vi "Pulse Measurement.vi"(0 "session":T3={"3620 session"=refnum, "tx baseband session"={"3610 session"={"VISA resource name"="", "Address Space"=1, "window_offset"=0, "register_addresses"={"MM based Registers"={"Revision"=0, "OldestCompatRev"=0, "signature"=0, "scratch"=0, "LedControl"=0, "BoardHwRev"=0, "BoardControl"=0, "ThermalStatus"=0, "BasebandStatus"=0, "BasebandControl"=0, "BasebandAuxSetup"=0, "BasebandAuxStatus"=0, "LmkSyncOutSetup"=0, " AdcSyncOutSetup"=0, " InjSyncOutSetup"=0, " PxiTrig0OutSetup"=0, " PxiTrig1OutSetup"=0, " PxiTrig2OutSetup"=0, " PxiTrig3OutSetup"=0, " PxiTrig4OutSetup"=0, " PxiTrig5OutSetup"=0, " PxiTrig6OutSetup"=0, " PxiTrig7OutSetup"=0}, "CPLD based Registers"={"SlaveSignature"=0, "SlaveRevision"=0, "SlaveOldestCompatRev"=0, "SlaveScratch"=0, "SlaveSetup"=0, "SlaveStatus"=0, "IDacReg_offset"=0, "LMKRegGrp0_offset"=0, "QDacReg_offset"=0, "BrdTempSensorVal"=0, "TempSensorPowerDown"=0, "GPIOReg_offset"=0, "IAdcReg_offset"=0, "QAdcReg_offset"=0, "LMKRegGrp1_offset"=0, "QadcTempSensorVal"=0, "IadcTempSensorVal"=0, "RevisionReg"=0, "VcxoReg"=0, "CpldStatusReg"=0, "PowerReg"=0, "VBiasEnReg"=0, "ExtRefOeReg"=0, "QdacCtrlReg"=0, "QdacStatusReg"=0, "IdacCtrlReg"=0, "IdacStatusReg"=0, "QdacJtagIn"=0, "QdacJtagOut"=0, "IdacJtagIn"=0, "IdacJtagOut"=0, "IqDcSetupReg"=0, "QadcStatusReg"=0, "IadcStatusReg"=0, "BrdSetupReg"=0, "IqDcRevisionReg"=0, "PllStatusReg"=0, "EndpointScratchReg"=0, "AdcSyncCfgReg"=0, "IqCardOpampReg"=0}, "CPLD Register Offset"=0, "MM  Register Offset"=0, " PxiTrig0OutSetup"=0}, "required_MM_fpga_version"={"signature"=0, "hardware"=0, "current revision"=0, "oldest revision"=0}, "CPLD Oldest Compat Version "={"hardware"=0, "CPLD firmware"=0}, "MM_FPGA_image_location"="", "is_init"=FALSE, "card_type"=enum."ADC", "DacLmkConfigFileName"="", "AdcLmkConfigFileName"="", "AdcConfigFileName"="", "DacConfigFileName_RevA"="", "DacConfigFileName_RevB"="", "Mulde hardware revision"=0, "bypass DAC PLL\n"=FALSE, "IQ Card Revision"=enum."RevA", "board capability"={"baseband sync"=enum."no baseband sync"}}, "7902 reference"=refnum}, "rx baseband session"={"3630 session"={"VISA resource name"="", "Address Space"=1, "window_offset"=0, "register_addresses"={"MM based Registers"={"Revision"=0, "OldestCompatRev"=0, "signature"=0, "scratch"=0, "LedControl"=0, "BoardHwRev"=0, "BoardControl"=0, "ThermalStatus"=0, "BasebandStatus"=0, "BasebandControl"=0, "BasebandAuxSetup"=0, "BasebandAuxStatus"=0, "LmkSyncOutSetup"=0, " AdcSyncOutSetup"=0, " InjSyncOutSetup"=0, " PxiTrig0OutSetup"=0, " PxiTrig1OutSetup"=0, " PxiTrig2OutSetup"=0, " PxiTrig3OutSetup"=0, " PxiTrig4OutSetup"=0, " PxiTrig5OutSetup"=0, " PxiTrig6OutSetup"=0, " PxiTrig7OutSetup"=0}, "CPLD based Registers"={"SlaveSignature"=0, "SlaveRevision"=0, "SlaveOldestCompatRev"=0, "SlaveScratch"=0, "SlaveSetup"=0, "SlaveStatus"=0, "IDacReg_offset"=0, "LMKRegGrp0_offset"=0, "QDacReg_offset"=0, "BrdTempSensorVal"=0, "TempSensorPowerDown"=0, "GPIOReg_offset"=0, "IAdcReg_offset"=0, "QAdcReg_offset"=0, "LMKRegGrp1_offset"=0, "QadcTempSensorVal"=0, "IadcTempSensorVal"=0, "RevisionReg"=0, "VcxoReg"=0, "CpldStatusReg"=0, "PowerReg"=0, "VBiasEnReg"=0, "ExtRefOeReg"=0, "QdacCtrlReg"=0, "QdacStatusReg"=0, "IdacCtrlReg"=0, "IdacStatusReg"=0, "QdacJtagIn"=0, "QdacJtagOut"=0, "IdacJtagIn"=0, "IdacJtagOut"=0, "IqDcSetupReg"=0, "QadcStatusReg"=0, "IadcStatusReg"=0, "BrdSetupReg"=0, "IqDcRevisionReg"=0, "PllStatusReg"=0, "EndpointScratchReg"=0, "AdcSyncCfgReg"=0, "IqCardOpampReg"=0}, "CPLD Register Offset"=0, "MM  Register Offset"=0, " PxiTrig0OutSetup"=0}, "required_MM_fpga_version"={"signature"=0, "hardware"=0, "current revision"=0, "oldest revision"=0}, "CPLD Oldest Compat Version "={"hardware"=0, "CPLD firmware"=0}, "MM_FPGA_image_location"="", "is_init"=FALSE, "card_type"=enum."ADC", "DacLmkConfigFileName"="", "AdcLmkConfigFileName"="", "AdcConfigFileName"="", "DacConfigFileName_RevA"="", "DacConfigFileName_RevB"="", "Mulde hardware revision"=0, "bypass DAC PLL\n"=FALSE, "IQ Card Revision"=enum."RevA", "board capability"={"baseband sync"=enum."no baseband sync"}}, "7902 reference"=refnum}, "tx gain (dB)"=0.0, "rx gain (dB)"=0.0, "hardware configuration"={"direction"=enum."Transceiver", "baseband only"=FALSE}, "gain ranging"=[], "pxi trigger bus information"={"chassis resource name"="", "7902R (TX)"=0, "3610 (TX)"=0, "3620 (IF)"=0, "3630 (RX)"=0, "7902R (RX)"=0}} {"rx baseband session"."3630 session"."Address Space" items=["VXI/VME A16"=1, "VXI/VME A24"=2, "VXI/VME A32"=3, "VXI/VME A64"=4, "PXI Memory Allocations"=9, "PXI Configuration"=10, "PXI BAR0"=11, "PXI BAR1"=12, "PXI BAR2"=13, "PXI BAR3"=14, "PXI BAR4"=15, "PXI BAR5"=16]; "tx baseband session"."3610 session"."Address Space" items=["VXI/VME A16"=1, "VXI/VME A24"=2, "VXI/VME A32"=3, "VXI/VME A64"=4, "PXI Memory Allocations"=9, "PXI Configuration"=10, "PXI BAR0"=11, "PXI BAR1"=12, "PXI BAR2"=13, "PXI BAR3"=14, "PXI BAR4"=15, "PXI BAR5"=16]}, 11 "error in":errorcluster) -> (4 "session out":T3={"3620 session"=refnum, "tx baseband session"={"3610 session"={"VISA resource name"="", "Address Space"=1, "window_offset"=0, "register_addresses"={"MM based Registers"={"Revision"=0, "OldestCompatRev"=0, "signature"=0, "scratch"=0, "LedControl"=0, "BoardHwRev"=0, "BoardControl"=0, "ThermalStatus"=0, "BasebandStatus"=0, "BasebandControl"=0, "BasebandAuxSetup"=0, "BasebandAuxStatus"=0, "LmkSyncOutSetup"=0, " AdcSyncOutSetup"=0, " InjSyncOutSetup"=0, " PxiTrig0OutSetup"=0, " PxiTrig1OutSetup"=0, " PxiTrig2OutSetup"=0, " PxiTrig3OutSetup"=0, " PxiTrig4OutSetup"=0, " PxiTrig5OutSetup"=0, " PxiTrig6OutSetup"=0, " PxiTrig7OutSetup"=0}, "CPLD based Registers"={"SlaveSignature"=0, "SlaveRevision"=0, "SlaveOldestCompatRev"=0, "SlaveScratch"=0, "SlaveSetup"=0, "SlaveStatus"=0, "IDacReg_offset"=0, "LMKRegGrp0_offset"=0, "QDacReg_offset"=0, "BrdTempSensorVal"=0, "TempSensorPowerDown"=0, "GPIOReg_offset"=0, "IAdcReg_offset"=0, "QAdcReg_offset"=0, "LMKRegGrp1_offset"=0, "QadcTempSensorVal"=0, "IadcTempSensorVal"=0, "RevisionReg"=0, "VcxoReg"=0, "CpldStatusReg"=0, "PowerReg"=0, "VBiasEnReg"=0, "ExtRefOeReg"=0, "QdacCtrlReg"=0, "QdacStatusReg"=0, "IdacCtrlReg"=0, "IdacStatusReg"=0, "QdacJtagIn"=0, "QdacJtagOut"=0, "IdacJtagIn"=0, "IdacJtagOut"=0, "IqDcSetupReg"=0, "QadcStatusReg"=0, "IadcStatusReg"=0, "BrdSetupReg"=0, "IqDcRevisionReg"=0, "PllStatusReg"=0, "EndpointScratchReg"=0, "AdcSyncCfgReg"=0, "IqCardOpampReg"=0}, "CPLD Register Offset"=0, "MM  Register Offset"=0, " PxiTrig0OutSetup"=0}, "required_MM_fpga_version"={"signature"=0, "hardware"=0, "current revision"=0, "oldest revision"=0}, "CPLD Oldest Compat Version "={"hardware"=0, "CPLD firmware"=0}, "MM_FPGA_image_location"="", "is_init"=FALSE, "card_type"=enum."ADC", "DacLmkConfigFileName"="", "AdcLmkConfigFileName"="", "AdcConfigFileName"="", "DacConfigFileName_RevA"="", "DacConfigFileName_RevB"="", "Mulde hardware revision"=0, "bypass DAC PLL\n"=FALSE, "IQ Card Revision"=enum."RevA", "board capability"={"baseband sync"=enum."no baseband sync"}}, "7902 reference"=refnum}, "rx baseband session"={"3630 session"={"VISA resource name"="", "Address Space"=1, "window_offset"=0, "register_addresses"={"MM based Registers"={"Revision"=0, "OldestCompatRev"=0, "signature"=0, "scratch"=0, "LedControl"=0, "BoardHwRev"=0, "BoardControl"=0, "ThermalStatus"=0, "BasebandStatus"=0, "BasebandControl"=0, "BasebandAuxSetup"=0, "BasebandAuxStatus"=0, "LmkSyncOutSetup"=0, " AdcSyncOutSetup"=0, " InjSyncOutSetup"=0, " PxiTrig0OutSetup"=0, " PxiTrig1OutSetup"=0, " PxiTrig2OutSetup"=0, " PxiTrig3OutSetup"=0, " PxiTrig4OutSetup"=0, " PxiTrig5OutSetup"=0, " PxiTrig6OutSetup"=0, " PxiTrig7OutSetup"=0}, "CPLD based Registers"={"SlaveSignature"=0, "SlaveRevision"=0, "SlaveOldestCompatRev"=0, "SlaveScratch"=0, "SlaveSetup"=0, "SlaveStatus"=0, "IDacReg_offset"=0, "LMKRegGrp0_offset"=0, "QDacReg_offset"=0, "BrdTempSensorVal"=0, "TempSensorPowerDown"=0, "GPIOReg_offset"=0, "IAdcReg_offset"=0, "QAdcReg_offset"=0, "LMKRegGrp1_offset"=0, "QadcTempSensorVal"=0, "IadcTempSensorVal"=0, "RevisionReg"=0, "VcxoReg"=0, "CpldStatusReg"=0, "PowerReg"=0, "VBiasEnReg"=0, "ExtRefOeReg"=0, "QdacCtrlReg"=0, "QdacStatusReg"=0, "IdacCtrlReg"=0, "IdacStatusReg"=0, "QdacJtagIn"=0, "QdacJtagOut"=0, "IdacJtagIn"=0, "IdacJtagOut"=0, "IqDcSetupReg"=0, "QadcStatusReg"=0, "IadcStatusReg"=0, "BrdSetupReg"=0, "IqDcRevisionReg"=0, "PllStatusReg"=0, "EndpointScratchReg"=0, "AdcSyncCfgReg"=0, "IqCardOpampReg"=0}, "CPLD Register Offset"=0, "MM  Register Offset"=0, " PxiTrig0OutSetup"=0}, "required_MM_fpga_version"={"signature"=0, "hardware"=0, "current revision"=0, "oldest revision"=0}, "CPLD Oldest Compat Version "={"hardware"=0, "CPLD firmware"=0}, "MM_FPGA_image_location"="", "is_init"=FALSE, "card_type"=enum."ADC", "DacLmkConfigFileName"="", "AdcLmkConfigFileName"="", "AdcConfigFileName"="", "DacConfigFileName_RevA"="", "DacConfigFileName_RevB"="", "Mulde hardware revision"=0, "bypass DAC PLL\n"=FALSE, "IQ Card Revision"=enum."RevA", "board capability"={"baseband sync"=enum."no baseband sync"}}, "7902 reference"=refnum}, "tx gain (dB)"=0.0, "rx gain (dB)"=0.0, "hardware configuration"={"direction"=enum."Transceiver", "baseband only"=FALSE}, "gain ranging"=[], "pxi trigger bus information"={"chassis resource name"="", "7902R (TX)"=0, "3610 (TX)"=0, "3620 (IF)"=0, "3630 (RX)"=0, "7902R (RX)"=0}} {"rx baseband session"."3630 session"."Address Space" items=["VXI/VME A16"=1, "VXI/VME A24"=2, "VXI/VME A32"=3, "VXI/VME A64"=4, "PXI Memory Allocations"=9, "PXI Configuration"=10, "PXI BAR0"=11, "PXI BAR1"=12, "PXI BAR2"=13, "PXI BAR3"=14, "PXI BAR4"=15, "PXI BAR5"=16]; "tx baseband session"."3610 session"."Address Space" items=["VXI/VME A16"=1, "VXI/VME A24"=2, "VXI/VME A32"=3, "VXI/VME A64"=4, "PXI Memory Allocations"=9, "PXI Configuration"=10, "PXI BAR0"=11, "PXI BAR1"=12, "PXI BAR2"=13, "PXI BAR3"=14, "PXI BAR4"=15, "PXI BAR5"=16]}, 8 "channel":T1, 15 "error out":errorcluster)   [LabVIEW 2019]
uses:
  TypeDefs/Session.ctl
  <instrlib>/niMmWave/ni3620/Config/v1/Host/Public/High-Level/niMmWave Session.ctl
  <instrlib>/_niInstr/Register Bus/v0/Host/Public/Register Bus Session.ctl
  <instrlib>/_niInstr/Register Bus/v0/Host/Private/Session Data.ctl
  <instrlib>/niMmWave/ni3620/Config/v1/Host/Public/Typedefs/Board Information.ctl
  <instrlib>/niMmWave/ni3620/Config/v1/Host/Public/Typedefs/Hardware Revision.ctl
  <instrlib>/niMmWave/ni3620/Config/v1/Host/Public/Typedefs/Gain Mapping.ctl
  <instrlib>/niMmWave/ni3620/Config/v1/Host/Public/Typedefs/Correction Data.ctl
  <instrlib>/niMmWave/ni3620/Config/v1/Host/Public/Typedefs/Opera Characterization.ctl
  <instrlib>/niMmWave/ni3620/Config/v1/Host/Public/Corrections/Typedefs/Opera Characterization Main Header.ctl
  <instrlib>/niMmWave/ni3620/Config/v1/Host/Public/Corrections/Typedefs/Opera IF Board Information.ctl
  <instrlib>/niMmWave/ni3620/Config/v1/Host/Public/Corrections/Typedefs/Opera Characterization Instance Header.ctl
  <instrlib>/niMmWave/ni3620/Config/v1/Host/Public/Corrections/Typedefs/Opera Characterization Device Data Header.ctl
  <instrlib>/niMmWave/ni3620/Config/v1/Host/Public/Corrections/Typedefs/Opera LO Characterization Data Header.ctl
  <instrlib>/niMmWave/ni3620/Config/v1/Host/Public/Corrections/Typedefs/Opera IF Board Characterization Data Header.ctl
  <instrlib>/niMmWave/ni3620/Config/v1/Host/Public/Corrections/Typedefs/Opera Characterization Device Data.ctl
  <instrlib>/niMmWave/ni3620/Config/v1/Host/Public/Corrections/Typedefs/Opera LO2 Board Characterization Data.ctl
  <instrlib>/niMmWave/ni3620/Config/v1/Host/Public/Corrections/Typedefs/Opera LO Characterization Data.ctl
  <instrlib>/niMmWave/ni3620/Config/v1/Host/Public/Corrections/Typedefs/Opera IF Board Characterization Data.ctl
  <instrlib>/niMmWave/ni3620/Config/v1/Host/Public/Corrections/Typedefs/Opera IQ Impairment Data.ctl
  <instrlib>/niMmWave/ni3620/Config/v1/Host/Public/Typedefs/mmWave Adapter Session Data.ctl
  <instrlib>/niMmWave/ni3620/Config/v1/Host/Public/Typedefs/mmWave Adapter Data.ctl
  <instrlib>/niMmWave/ni3620/Config/v1/Host/Public/Typedefs/mmWave Adapter 2.ctl
  <instrlib>/niMmWave/ni3620/Config/v1/Shared/Typedefs/Subsystem ID.ctl
  <instrlib>/niMmWave/ni3620/Config/v1/Host/Public/Typedefs/mmWave Adapter Channel Information.ctl
  <instrlib>/niMmWave/ni3620/Config/v1/Host/Public/Typedefs/Temperature Coefficients.ctl
  <instrlib>/niMmWave/ni3620/Config/v1/Host/Public/Typedefs/mmWave Characterization.ctl
  <instrlib>/niMmWave/ni3620/Config/v1/Host/Public/Corrections/Typedefs/mmWave Characterization Main Header.ctl
  <instrlib>/niMmWave/ni3620/Config/v1/Host/Public/Corrections/Typedefs/mmWave Characterization Instance Header.ctl
  <instrlib>/niMmWave/ni3620/Config/v1/Host/Public/Typedefs/Session Cache.ctl
  <instrlib>/niMmWave/ni3620/Config/v1/Host/Public/Typedefs/LO2 settings cache.ctl
  <instrlib>/niMmWave/ni3620/Config/v1/Host/Public/Typedefs/LO2 source.ctl
  <instrlib>/niMmWave/ni3620/Config/v1/Host/Public/Typedefs/Desired and Coerced.ctl
  <instrlib>/niMmWave/ni3620/Config/v1/Host/Public/Typedefs/Export cache.ctl
  <instrlib>/niMmWave/ni3620/Config/v1/Host/Public/Typedefs/Path cache.ctl
  <instrlib>/niMmWave/ni3620/Config/v1/Host/Public/Typedefs/Daughterboard Type.ctl
  <instrlib>/niMmWave/ni3620/Config/v1/Host/Public/Typedefs/LO1 settings cache.ctl
  <instrlib>/niMmWave/ni3620/Config/v1/Host/Public/Typedefs/LO1 Source.ctl
  <instrlib>/niMmWave/ni3620/Config/v1/Host/Public/Typedefs/mmWave export cache.ctl
  <instrlib>/niMmWave/ni3620/Config/v1/Host/Private/Board/LO2/LO2 Board Configuration Cache.ctl
  <instrlib>/niMmWave/ni3620/Config/v1/Host/Public/Typedefs/reference clock routing settings.ctl
  <instrlib>/niMmWave/ni3620/Config/v1/Host/Public/Typedefs/LO2 routing settings.ctl
  <instrlib>/niMmWave/ni3620/Config/v1/Host/Private/Board/LO1/LO1 Board Configuration Cache.ctl
  <instrlib>/niMmWave/ni3620/Config/v1/Host/Public/Typedefs/LO1 source settings.ctl
  <instrlib>/niMmWave/ni3620/Config/v1/Host/Public/Typedefs/LO1 export settings.ctl
  <instrlib>/niMmWave/ni3620/Config/v1/Host/Public/Typedefs/LO1 mmWave settings.ctl
  TypeDefs/Tx Baseband Session.ctl
  <instrlib>/niMmWave/ni3610 and ni3630/controls/public/Main Settings.ctl
  <vilib>/Instr/_visa.llb/VISA Register Access Address Space.ctl
  <instrlib>/niMmWave/ni3610 and ni3630/controls/public/Register Adresses.ctl
  <instrlib>/niMmWave/ni3610 and ni3630/controls/public/Base Card Type.ctl
  <instrlib>/niMmWave/ni3610 and ni3630/controls/private/IQ Card Revision.ctl
  <instrlib>/niMmWave/ni3610 and ni3630/controls/public/Board Capability.ctl
  TypeDefs/Blank FPGA Reference.ctl
  TypeDefs/Rx Baseband Session.ctl
  TypeDefs/Hardware Configuration.ctl
  TypeDefs/Direction.ctl
  TypeDefs/Gain Ranging.ctl
  TypeDefs/PXI Trigger Bus Info.ctl
  TypeDefs/TX FPGA Reference.ctl
  <vilib>/Analysis/4window.llb/windowTd.ctl
  <vilib>/Analysis/1siggen.llb/Ramp Pattern by Samples.vi
  <vilib>/Analysis/2dsp.llb/Complex FFT.vi
  <vilib>/Analysis/baseanly.llb/Mean (DBL).vi
  <vilib>/Utility/error.llb/Error Cluster From Error Code.vi
  <vilib>/rvi/errors/niLvFpgaAdjustHostInterfaceError.vi
  <vilib>/Analysis/0measdsp.llb/Scaled Time Domain Window (CDB).vi
  <vilib>/Analysis/6fits.llb/1D B-Spline Fit.vi
  <vilib>/rvi/interface/nirviReadWriteControl/nirviReadWriteControl.xnode
  <vilib>/Analysis/NI_AALBase.lvlib
  NiFpgaLv.dll
  <vilib>/rvi/interface/Simulation/niFpgaSimulationCallBeginRW.vi
  <vilib>/Analysis/NI_AALPro.lvlib
  <instrlib>/_niInstr/Register Bus/v0/Host/niInstr Register Bus v0 Host.lvlib
  <instrlib>/niMmWave/ni3610 and ni3630/ni3610_and_ni3630_Driver_Lib.lvlib
  <instrlib>/niMmWave/ni3620/Config/v1/Host/niMmWave Config v1 Host.lvlib
  <instrlib>/niMmWave/ni3620/Config/v1/Shared/niMmWave Config v1 Shared.lvlib
panel:
  out "magnitude":T2(graph)
  out "phase":T2(graph)
  out "phase raw":cluster{"Ramp Pattern":dbl[], dbl[]}[](graph)
  out "magnitude raw":cluster{"Ramp Pattern":dbl[], dbl[]}[](graph)
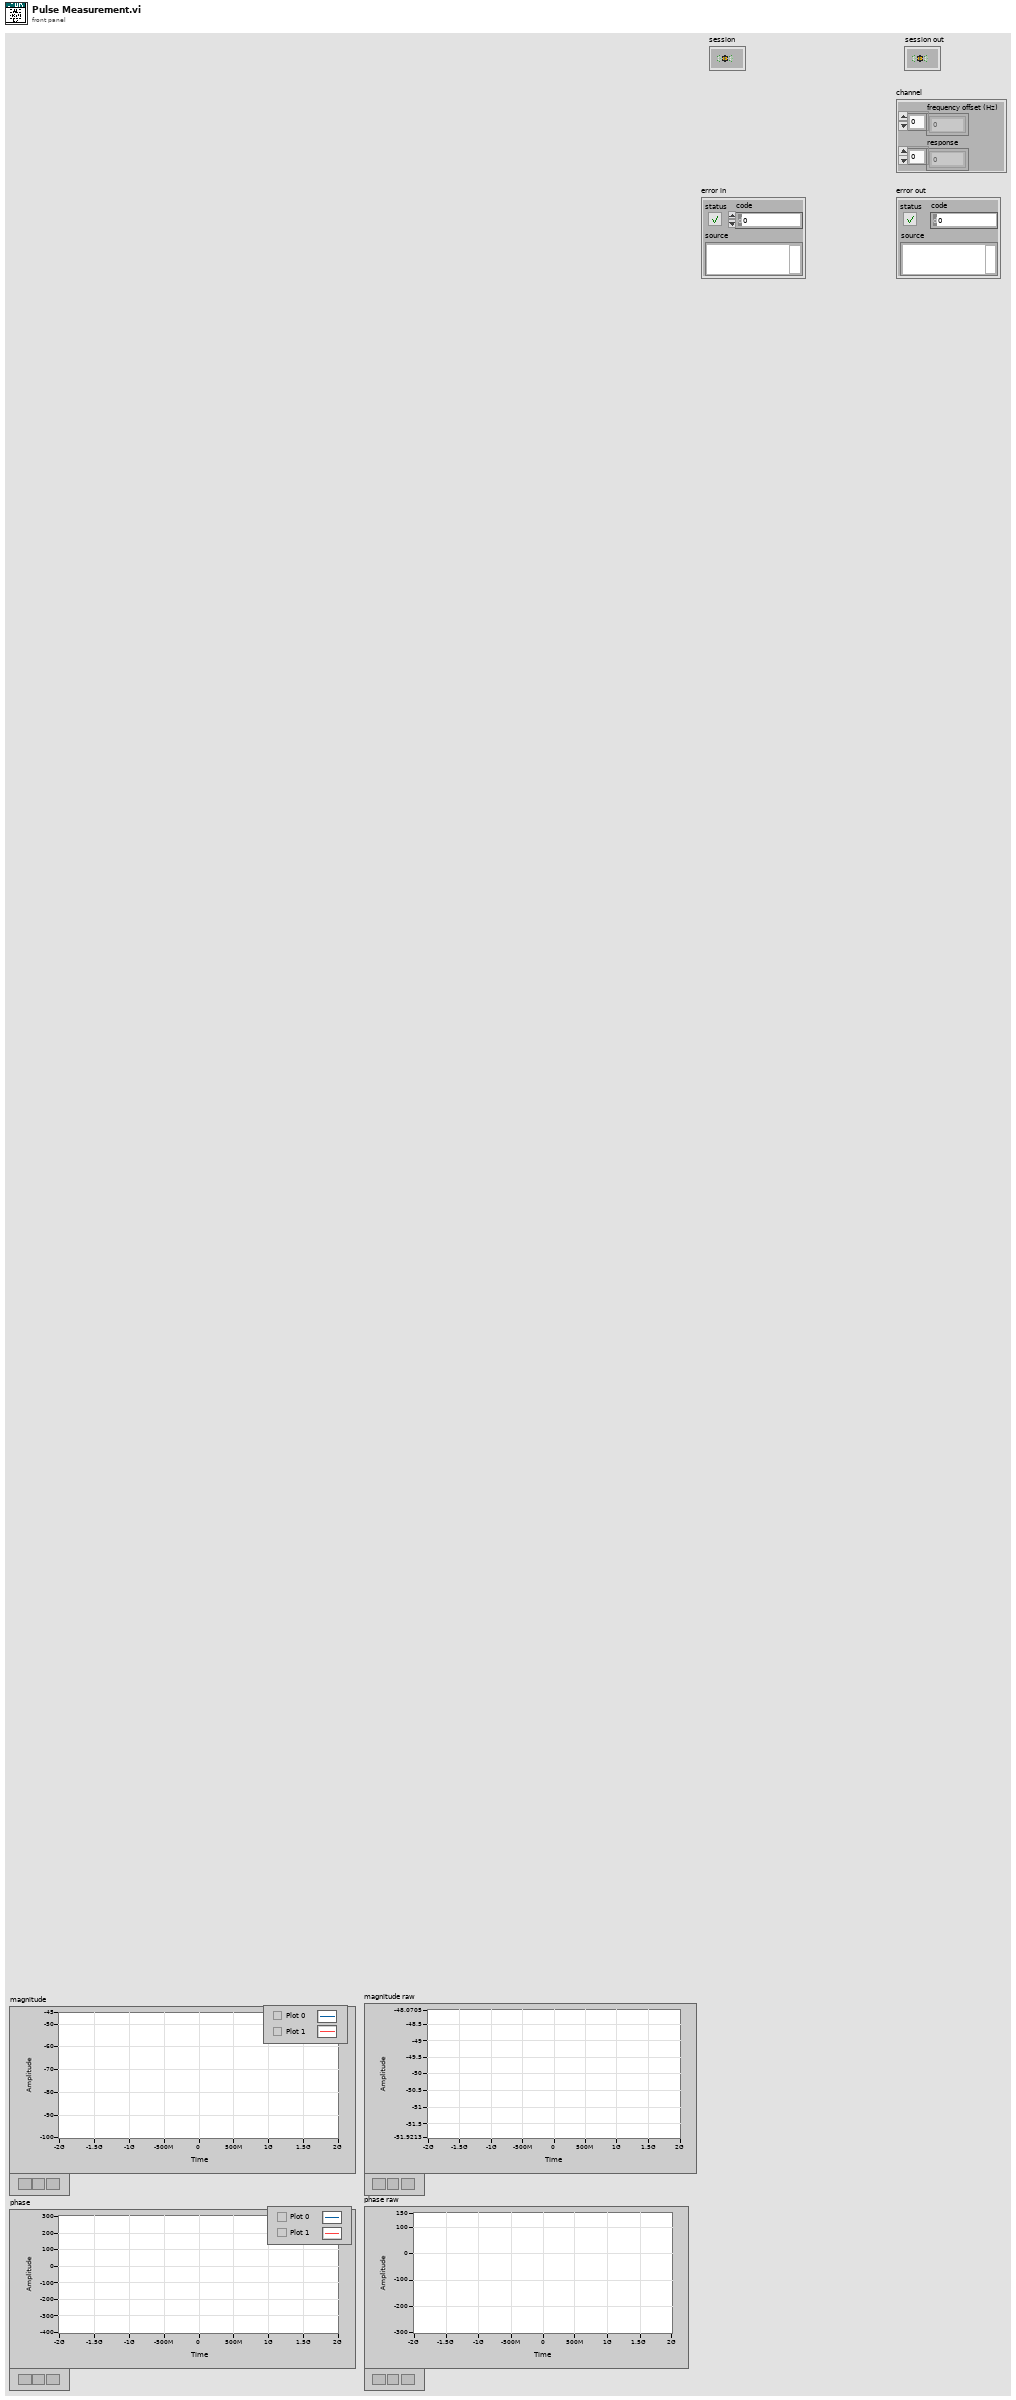
[diagram p1: front panel]
types:
  T1 = cluster{"frequency offset (Hz)":dbl[], "response":cdb[]}
  T2 = cluster{"Ramp Pattern":dbl[], "Best BSpline Fit Y":dbl[]}[]
  T3 = typedef "Session.ctl" = cluster{"3620 session":refnum<queue>, "tx baseband session":T4, "rx baseband session":T12, "tx gain (dB)":dbl, "rx gain (dB)":dbl, "hardware configuration":T13, "gain ranging":T15[], "pxi trigger bus information":T16}
  T4 = typedef "Tx Baseband Session.ctl" = cluster{"3610 session":T5, "7902 reference":T11}
  T5 = typedef "ni3610_and_ni3630_Driver_Lib.lvlib/Main Settings.ctl" = cluster{"VISA resource name":refnum<visa-resource-name>, "Address Space":T6, "window_offset":u32, "register_addresses":T7, "required_MM_fpga_version":cluster{"signature":u32, "hardware":u32, "current revision":u32, "oldest revision":u32}, "CPLD Oldest Compat Version ":cluster{"hardware":u32, "CPLD firmware":u32}, "MM_FPGA_image_location":string, "is_init":bool, "card_type":T8, "DacLmkConfigFileName":string, "AdcLmkConfigFileName":string, "AdcConfigFileName":string, "DacConfigFileName_RevA":string, "DacConfigFileName_RevB":string, "Mulde hardware revision":u8, "bypass DAC PLL\n":bool, "IQ Card Revision":T9, "board capability":T10}
  T6 = typedef "VISA Register Access Address Space.ctl" = u16
  T7 = typedef "ni3610_and_ni3630_Driver_Lib.lvlib/Register Adresses.ctl" = cluster{"MM based Registers":cluster{"Revision":u32, "OldestCompatRev":u32, "signature":u32, "scratch":u32, "LedControl":u32, "BoardHwRev":u32, "BoardControl":u32, "ThermalStatus":u32, "BasebandStatus":u32, "BasebandControl":u32, "BasebandAuxSetup":u32, "BasebandAuxStatus":u32, "LmkSyncOutSetup":u32, " AdcSyncOutSetup":u32, " InjSyncOutSetup":u32, " PxiTrig0OutSetup":u32, " PxiTrig1OutSetup":u32, " PxiTrig2OutSetup":u32, " PxiTrig3OutSetup":u32, " PxiTrig4OutSetup":u32, " PxiTrig5OutSetup":u32, " PxiTrig6OutSetup":u32, " PxiTrig7OutSetup":u32}, "CPLD based Registers":cluster{"SlaveSignature":u32, "SlaveRevision":u32, "SlaveOldestCompatRev":u32, "SlaveScratch":u32, "SlaveSetup":u32, "SlaveStatus":u32, "IDacReg_offset":u32, "LMKRegGrp0_offset":u32, "QDacReg_offset":u32, "BrdTempSensorVal":u32, "TempSensorPowerDown":u32, "GPIOReg_offset":u32, "IAdcReg_offset":u32, "QAdcReg_offset":u32, "LMKRegGrp1_offset":u32, "QadcTempSensorVal":u32, "IadcTempSensorVal":u32, "RevisionReg":u32, "VcxoReg":u32, "CpldStatusReg":u32, "PowerReg":u32, "VBiasEnReg":u32, "ExtRefOeReg":u32, "QdacCtrlReg":u32, "QdacStatusReg":u32, "IdacCtrlReg":u32, "IdacStatusReg":u32, "QdacJtagIn":u32, "QdacJtagOut":u32, "IdacJtagIn":u32, "IdacJtagOut":u32, "IqDcSetupReg":u32, "QadcStatusReg":u32, "IadcStatusReg":u32, "BrdSetupReg":u32, "IqDcRevisionReg":u32, "PllStatusReg":u32, "EndpointScratchReg":u32, "AdcSyncCfgReg":u32, "IqCardOpampReg":u32}, "CPLD Register Offset":u32, "MM  Register Offset":u32, " PxiTrig0OutSetup":u32}
  T8 = typedef "ni3610_and_ni3630_Driver_Lib.lvlib/Base Card Type.ctl" = enum16{"unspecified", "ADC", "DAC"}
  T9 = typedef "ni3610_and_ni3630_Driver_Lib.lvlib/IQ Card Revision.ctl" = enum16{"RevA", "RevB", "RevC", "RevD"}
  T10 = typedef "ni3610_and_ni3630_Driver_Lib.lvlib/Board Capability.ctl" = cluster{"baseband sync":enum16{"no baseband sync", "baseband sync"}}
  T11 = typedef "Blank FPGA Reference.ctl" = refnum<k20>
  T12 = typedef "Rx Baseband Session.ctl" = cluster{"3630 session":T5, "7902 reference":T11}
  T13 = typedef "Hardware Configuration.ctl" = cluster{"direction":T14, "baseband only":bool}
  T14 = typedef "Direction.ctl" = enum16{"Transceiver", "Receiver", "Transmitter"}
  T15 = typedef "Gain Ranging.ctl" = cluster{"gain ranging active scope":string, "gain ranging stream session":refnum<k20>}
  T16 = typedef "PXI Trigger Bus Info.ctl" = cluster{"chassis resource name":refnum<visa-resource-name>, "7902R (TX)":i16, "3610 (TX)":i16, "3620 (IF)":i16, "3630 (RX)":i16, "7902R (RX)":i16}
  T17 = enum16{"Pass Through", "Tone", "Pulse", "Disable"}
  T18 = cluster{"frequency":u32, "gain":fxp<+/-,18,1>, "width":u8}
  T19 = typedef "TX FPGA Reference.ctl" = refnum<k20>
  T20 = typedef "Constants.ctl" = cluster{"data clock rate (Hz)":dbl, "sample rate (Hz)":dbl, "sample rate selector string":string, "default tx bitfile path":path, "default rx bitfile path":path, "default proc bitfile path":path}
  T21 = cluster{"generation select":enum16{"Pass Through", "Tone", "Pulse", "Disable"}, "tone parameters":cluster{"frequency":fxp<+/-,48,0>, "gain":fxp<+/-,18,1>}, "pulse parameters":cluster{"frequency":u32, "gain":fxp<+/-,18,1>, "width":u8}}
  T22 = typedef "NI_AALPro.lvlib/windowTd.ctl" = u32
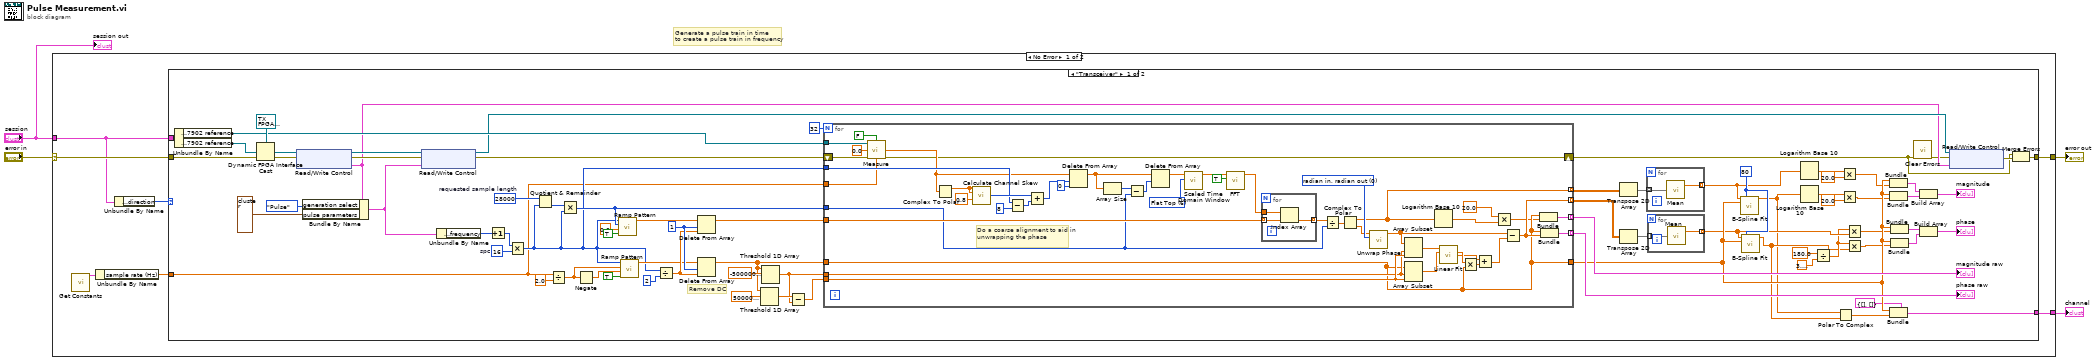
[diagram p0: block diagram]
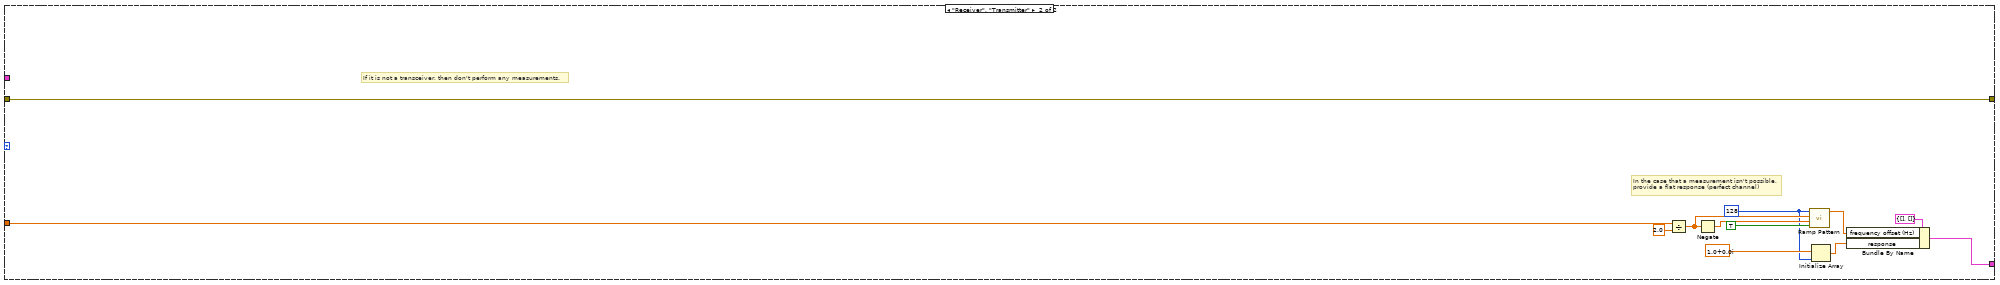
[diagram p2: hidden frame]
diagram:
  # "Generate a pulse train in time\nto create a pulse train in frequency"
  n1 = case shown="No Error" "error in" {
    selector: "error in" -> [w10 w154]
    tunnel: "session" -> [w8 _]
    tunnel: [w9 w154] -> w3
    tunnel: [w11 _] -> w1
    frame No Error {
      n2 = call "Get Constants.vi"() -> ("constants"=w6:T20)  [unwired: 15 in]
      n3 = Unbundle By Name(w6) -> ("sample rate (Hz)"=w5:dbl)
      n4 = Unbundle By Name(w8) -> ("hardware configuration.direction"=w7:T14)
      n5 = case shown="\"Transceiver\"" w7 {
        tunnel: w8 -> [w88 _]
        tunnel: [w42 w143] -> w11
        tunnel: w10 -> [w38 w153]
        tunnel: [w16 w153] -> w9
        tunnel: w5 -> [w12 w142]
        frame "Transceiver" {
          w51 = 80 ("# of control points")
          w64 = 28000  # requested sample length
          w68 = 1 ("length")
          w83 = u32 16  # spc
          # "Remove DC"
          n6 = Unbundle By Name(w88) -> ("rx baseband session.7902 reference"=w60:T11, "tx baseband session.7902 reference"=w86:T11)
          n7 = Dynamic FPGA Interface Cast(Session In=T19 refnum ("Refnum in"), Type=w86) -> (Session Out=w40:T19)
          n8 = xnode "Read/Write Control"("FPGA VI Reference In"=w40, "error in"=w38) -> ("FPGA VI Reference Out"=w39:T19, "error out"=w37:errorcluster, "cal.generation"=w32:T21)
          n9 = Bundle By Name(cluster=w32, "generation select"=T17."Pulse", "pulse parameters"=T18 {"frequency"=10, "gain"=0.5, "width"=1}) -> (w34:T21)
          n10 = xnode "Read/Write Control"("FPGA VI Reference In"=w39, "error in"=w37, "cal.generation"=w34) -> ("FPGA VI Reference Out"=w33:T19, "error out"=w58:errorcluster)
          n11 = Unbundle By Name(w34) -> ("pulse parameters.frequency"=w85:u32)
          n12 = Increment(x=w85) -> (x+1=w84:u32)
          n13 = Multiply(x=w84, y=w83) -> (x*y=w59:u32)
          n14 = Quotient & Remainder(x=w64, y=w59) -> (floor(x/y)=w65:u32)  [unwired: 1 out]
          n15 = Divide(x=w12, y=2.0) -> (x/y=w80:dbl)
          n16 = Multiply(x=w65, y=w59) -> (x*y=w63:u32)
          n17 = Negate(x=w80) -> (-x=w81:dbl)
          n18 = call-poly <vilib>:"Ramp Pattern.vi"("exclude end?"=TRUE, "start"=0.0, "end"=w63, "samples"=w59) -> ("Ramp Pattern"=w70:dbl[])  [unwired: 6 in, 1 out]
          n19 = call-poly <vilib>:"Ramp Pattern.vi"("exclude end?"=TRUE, "start"=w81, "end"=w80, "samples"=w59) -> ("Ramp Pattern"=w66:dbl[])  [unwired: 6 in, 1 out]
          n20 = Divide(x=w59, y=2) -> (x/y=w67:dbl)
          n21 = Delete From Array(array=w70, length=w68, index=w67) -> (array with subset deleted=w69:dbl[])  [unwired: 1 out]
          n22 = Delete From Array(array=w66, length=w68, index=w67) -> (array with subset deleted=w49:dbl[])  [unwired: 1 out]
          n23 = Threshold 1D Array(2:500000000.0 ("threshold y"), 3:w49) -> (0:w47:dbl)  [unwired: 1 in]
          n24 = Threshold 1D Array(2:-500000000.0 ("threshold y"), 3:w49) -> (0:w45:dbl)  [unwired: 1 in]
          n25 = Subtract(x=w47, y=w45) -> (x-y=w46:dbl)
          n26 = for {
            N: 32 ("Numeric 2") -> [_]
            tunnel: [w111] -> w77 mode=indexing
            tunnel: w49 -> [w98]
            tunnel: w59 -> [w114]
            tunnel: [w98] -> w43
            tunnel: [w92] -> w74 mode=indexing
            tunnel: w69 -> [w123]
            tunnel: [w130] -> w61 mode=indexing
            tunnel: [w124] -> w62 mode=indexing
            tunnel: w63 -> [w113]
            tunnel: w60 -> [w109]
            shift-right: [w107] -> w13
            shift-left: w58 -> [w108]
            tunnel: w12 -> [w106]
            tunnel: w46 -> [w100]
            tunnel: w45 -> [w99]
            w112 = T22 6 items=["Rectangle"=0, "Hanning"=1, "Hamming"=2, "Blackman-Harris"=3, "Exact Blackman"=4, "Blackman"=5, "Flat Top"=6, "4 Term B-Harris "=7, "7 Term B-Harris"=8, "Low Sidelobe"=9, "Blackman Nuttall"=11, "Triangle"=30, "Bartlett-Hanning"=31, "Bohman"=32, "Parzen"=33, "Welch"=34, "Kaiser"=60, "Dolph-Chebyshev"=61, "Gaussian"=62] ("window")
            w125 = 0 items=["radian in, radian out", "radian in, degree out", "degree in, degree out", "degree in, radian out"] ("phase unit")
            # "Do a coarse alignment to aid in unwrapping the phase"
            n27 = call "Measure.vi"("rx fpga reference in"=w109, "calculate measurements"=FALSE, "frequency (Hz)"=0.0, "error in"=w108, "IQ rate"=w106) -> ("raw data"=w110:cdb[], "error out"=w107:errorcluster)  [unwired: 7 in, 2 out]
            n28 = Complex To Polar(r * e^(i*theta)=w110) -> (r=w116:dbl[])  [unwired: 1 out]
            n29 = call "Calculate Channel Skew.vi"("channel 1"=w116, "channel 2"=w116, "threshold"=0.8) -> ("falling edge index"=w121:i32)  [unwired: 10 in, 2 out]
            n30 = Subtract(x=w114, y=8) -> (x-y=w119:u32)
            n31 = Add(x=w121, y=w119) -> (x+y=w117:u32)
            n32 = Delete From Array(array=w110, length=w117, index=0) -> (array with subset deleted=w115:cdb[])  [unwired: 1 out]
            n33 = Array Size(array=w115) -> (size(s)=w133:i32)
            n34 = Subtract(x=w133, y=w113) -> (x-y=w132:u32)
            n35 = Delete From Array(array=w115, length=w132) -> (array with subset deleted=w126:cdb[])  [unwired: 1 in, 1 out]
            n36 = call-poly <vilib>:"Scaled Time Domain Window.vi"("window"=w112, "X"=w126) -> ("Windowed X"=w131:cdb[])  [unwired: 7 in, 2 out]
            n37 = call-poly <vilib>:"FFT.vi"("shift?"=TRUE, "X"=w131) -> ("FFT {X}"=w127:cdb[])  [unwired: 8 in, 1 out]
            n38 = for {
              tunnel: w123 -> [w137] mode=indexing
              tunnel: w127 -> [w136]
              tunnel: [w135] -> w129 mode=indexing
              n39 = Index Array(array=w136, index=w137) -> (element=w135:cdb)
            }
            n40 = Divide(x=w129, y=w113) -> (x/y=w128:cdb[])
            n41 = Complex To Polar(r * e^(i*theta)=w128) -> (r=w92:dbl[], theta=w93:dbl[])
            n42 = call <vilib>:"Unwrap Phase.vi"("phase unit"=w125, "Phase"=w93) -> ("Unwrapped Phase"=w103:dbl[])  [unwired: 8 in, 1 out]
            n43 = Array Subset(array=w103, index=w99, length=w100) -> (w102:dbl[])
            n44 = Array Subset(array=w98, index=w99, length=w100) -> (w101:dbl[])
            n45 = Logarithm Base 10(1:w92) -> (0:w91:dbl[])
            n46 = call <vilib>:"Linear Fit.vi"("Y"=w102, "X"=w101) -> ("slope"=w97:dbl, "intercept"=w95:dbl)  [unwired: 9 in, 3 out]
            n47 = Multiply(x=w97, y=w98) -> (x*y=w96:dbl[])
            n48 = Add(x=w95, y=w96) -> (x+y=w94:dbl[])
            n49 = Multiply(x=20.0, y=w91) -> (x*y=w89:dbl[])
            n50 = Subtract(x=w103, y=w94) -> (x-y=w111:dbl[])
            n51 = Bundle("Ramp Pattern"=w98, w89) -> (w130:cluster{"Ramp Pattern":dbl[], dbl[]})  [unwired: 1 in]
            n52 = Bundle("Ramp Pattern"=w98, w111) -> (w124:cluster{"Ramp Pattern":dbl[], dbl[]})  [unwired: 1 in]
          }
          "magnitude raw" <- w61
          "phase raw" <- w62
          n53 = Transpose 2D Array(2D array=w74) -> (transposed array=w75:dbl[][])
          n54 = Transpose 2D Array(2D array=w77) -> (transposed array=w76:dbl[][])
          n55 = for {
            tunnel: w75 -> [w141] mode=indexing
            tunnel: [w140] -> w23 mode=indexing
            n56 = call-poly <vilib>:"Mean.vi"("X"=w141) -> ("mean"=w140:dbl)  [unwired: 1 out]
          }
          n57 = for {
            tunnel: w76 -> [w139] mode=indexing
            tunnel: [w138] -> w29 mode=indexing
            n58 = call-poly <vilib>:"Mean.vi"("X"=w139) -> ("mean"=w138:dbl)  [unwired: 1 out]
          }
          n59 = call-poly <vilib>:"B-Spline Fit.vi"("Y"=w23, "# of control points"=w51, "X"=w43) -> ("Best BSpline Fit Y"=w18:dbl[])  [unwired: 9 in, 3 out]
          n60 = call-poly <vilib>:"B-Spline Fit.vi"("Y"=w29, "# of control points"=w51, "X"=w43) -> ("Best BSpline Fit Y"=w26:dbl[])  [unwired: 9 in, 3 out]
          n61 = Logarithm Base 10(1:w23) -> (0:w22:dbl[])
          n62 = Logarithm Base 10(1:w18) -> (0:w19:dbl[])
          n63 = Divide(x=180.0, y=3.141592653589793) -> (x/y=w27:dbl)
          n64 = Polar To Complex(1:w26, 2:w18) -> (0:w44:cdb[])
          n65 = Multiply(x=w22, y=20.0) -> (x*y=w21:dbl[])
          n66 = Multiply(x=w19, y=20.0) -> (x*y=w17:dbl[])
          n67 = Multiply(x=w27, y=w29) -> (x*y=w28:dbl[])
          n68 = Multiply(x=w27, y=w26) -> (x*y=w25:dbl[])
          n69 = Bundle("Ramp Pattern"=w43, w21) -> (w57:cluster{"Ramp Pattern":dbl[], dbl[]})  [unwired: 1 in]
          n70 = Bundle("Ramp Pattern"=w43, w17) -> (w56:cluster{"Ramp Pattern":dbl[], dbl[]})  [unwired: 1 in]
          n71 = Bundle(cluster=T1 {"frequency offset (Hz)"=[], "response"=[]} ("channel 2"), "frequency offset (Hz)"=w43, "response"=w44) -> (w42:T1)
          n72 = Bundle("Ramp Pattern"=w43, w28) -> (w54:cluster{"Ramp Pattern":dbl[], dbl[]})  [unwired: 1 in]
          n73 = Bundle("Ramp Pattern"=w43, w25) -> (w53:cluster{"Ramp Pattern":dbl[], dbl[]})  [unwired: 1 in]
          n74 = call <vilib>:"Clear Errors.vi"("error in (no error)"=w13) -> ("error out"=w15:errorcluster)  [unwired: 5 in, 1 out]
          n75 = Build Array(w57, w56) -> (→"magnitude":cluster{"Ramp Pattern":dbl[], dbl[]}[])
          n76 = Build Array(w54, w53) -> (→"phase":cluster{"Ramp Pattern":dbl[], dbl[]}[])
          n77 = xnode "Read/Write Control"("FPGA VI Reference In"=w33, "error in"=w15, "cal.generation"=w32) -> ("error out"=w14:errorcluster)  [unwired: 1 out]
          n78 = Merge Errors(w13, w14) -> (w16:errorcluster)
        }
        frame "Receiver", "Transmitter" {
          w144 = 128 ("samples")
          # "In the case that a measurement isn't possible,\nprovide a flat response (perfect channel)"
          # "If it is not a transceiver, then don't perform any measurements."
          n79 = Divide(x=w142, y=2.0) -> (x/y=w150:dbl)
          n80 = Negate(x=w150) -> (-x=w151:dbl)
          n81 = call-poly <vilib>:"Ramp Pattern.vi"("exclude end?"=TRUE, "start"=w151, "end"=w150, "samples"=w144) -> ("Ramp Pattern"=w147:dbl[])  [unwired: 6 in, 1 out]
          n82 = Initialize Array(cdb 1.0+0.0i, w144) -> (w145:cdb[])
          n83 = Bundle By Name(cluster=T1 {"frequency offset (Hz)"=[], "response"=[]} ("channel 2"), "frequency offset (Hz)"=w147, "response"=w145) -> (w143:T1)
        }
      }
    }
    frame Error {
    }
  }
  "error out" <- w3
  "channel" <- w1
  "session out" <- "session"
